vi "自动售货机.vi"() -> ()   [LabVIEW 2011]
panel:
  out "消费额":dbl
  out "投币金额":dbl=79.0
  in  "Tab Control":enum32{"售卖界面", "后台操作界面"}(tab)=enum."后台操作界面"
  out "出货信息":string
  out "显示金额":string
  in  "退币":bool
  in  "5角":bool
  in  "5元":bool
  in  "1元":bool
  in  "10元":bool
  out "果粒橙P":string="0元"
  out "营养快线P":string="0元"
  out "矿泉水P":string="0元"
  out "花生奶P":string="0元"
  out "绿茶P":string="0元"
  out "雪梨P":string="0元"
  in  "果粒橙":bool
  in  "营养快线":bool
  in  "矿泉水":bool
  in  "花生奶":bool
  in  "绿茶":bool
  in  "雪梨":bool
  out "红牛P":string="0元"
  out "八宝粥P":string="0元"
  out "王老吉P":string="0元"
  out "可乐P":string="0元"
  out "雪碧P":string="0元"
  out "百事P":string="0元"
  in  "红牛":bool
  in  "八宝粥":bool
  in  "王老吉":bool
  in  "可乐":bool
  in  "雪碧":bool
  in  "百事":bool
  in  "上货":bool
  in  "关闭售货机":bool
  in  "果粒橙单价":dbl=4.0
  in  "营养快线单价":dbl=3.5
  in  "矿泉水单价":dbl=1.5
  in  "花生奶单价":dbl=3.5
  in  "绿茶单价":dbl=2.5
  in  "雪梨单价":dbl=2.5
  in  "红牛单价":dbl=4.0
  in  "八宝粥单价":dbl=3.0
  in  "王老吉单价":dbl=3.0
  in  "可乐单价":dbl=2.0
  in  "雪碧单价":dbl=2.0
  in  "百事单价":dbl=2.0
  out "销售记录":string
  out "销售金额":string
  in  "果粒橙数量":i32=20
  in  "营养快线数量":i32=20
  in  "矿泉水数量":i32=20
  in  "花生奶数量":i32=20
  in  "绿茶数量":i32=20
  in  "雪梨数量":i32=20
  in  "红牛数量":i32=20
  in  "八宝粥数量":i32=20
  in  "王老吉数量":i32=20
  in  "可乐数量":i32=20
  in  "雪碧数量":i32=20
  in  "百事数量":i32=20
  # "实验中心"
  # "chn"
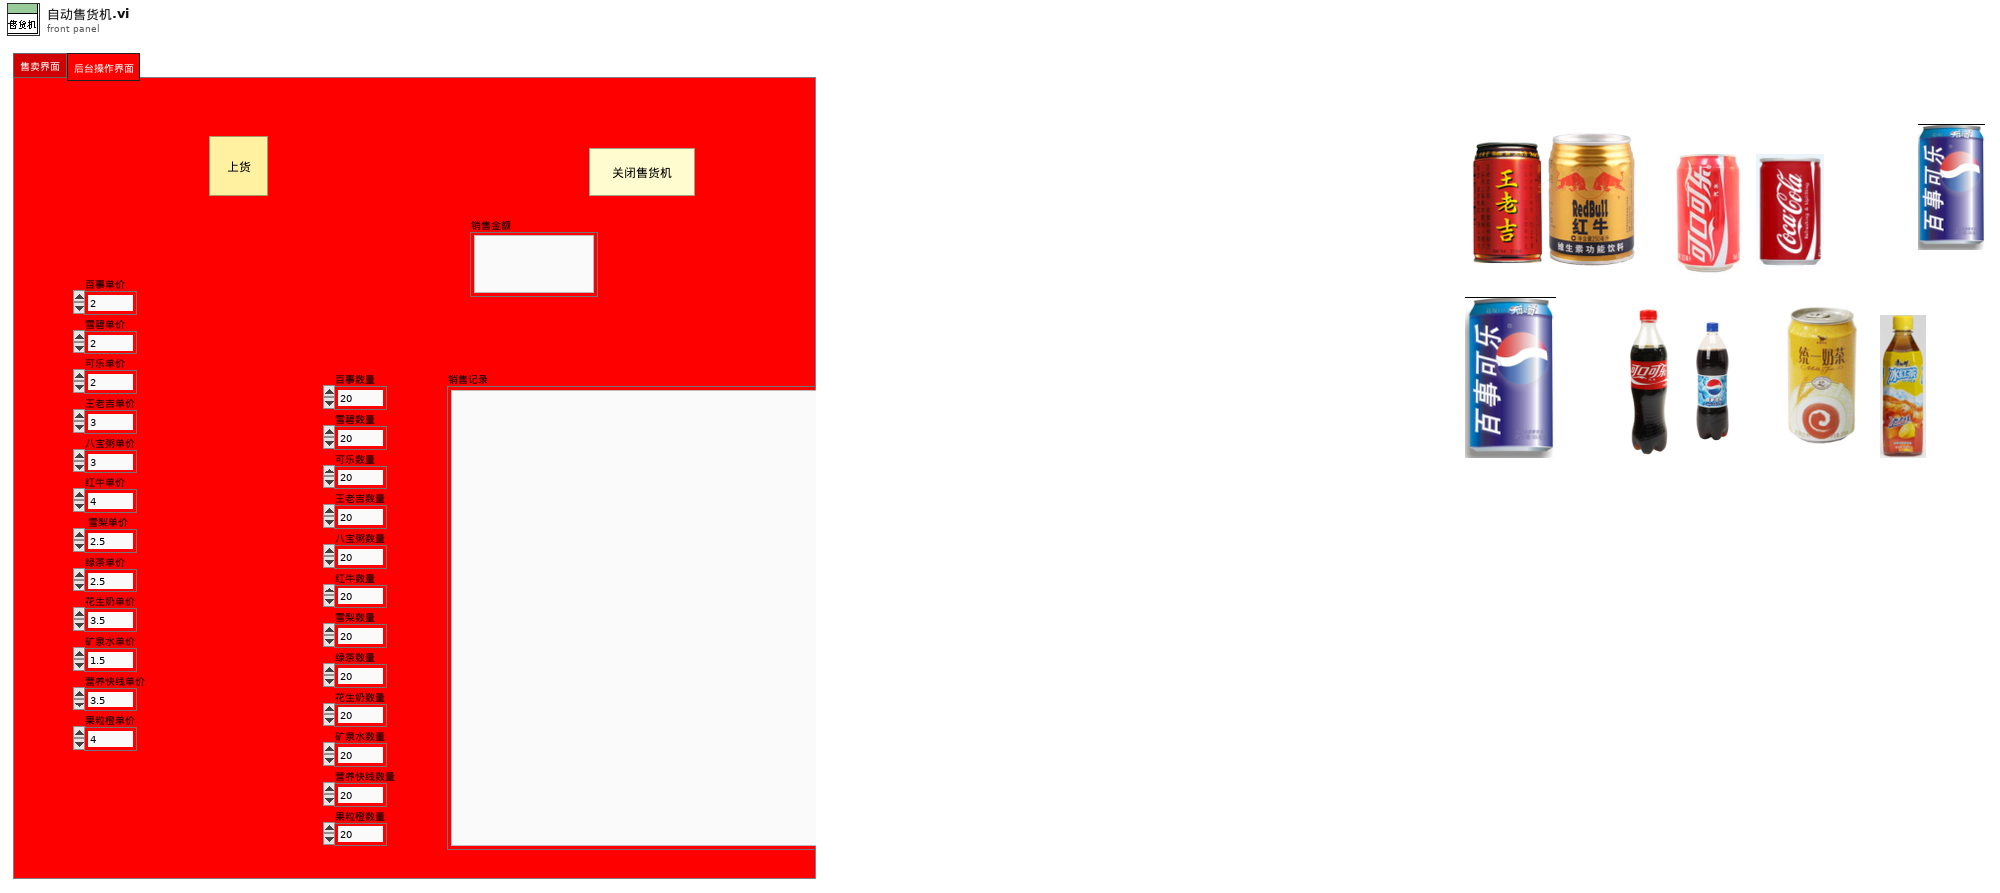
[diagram p1: front panel]
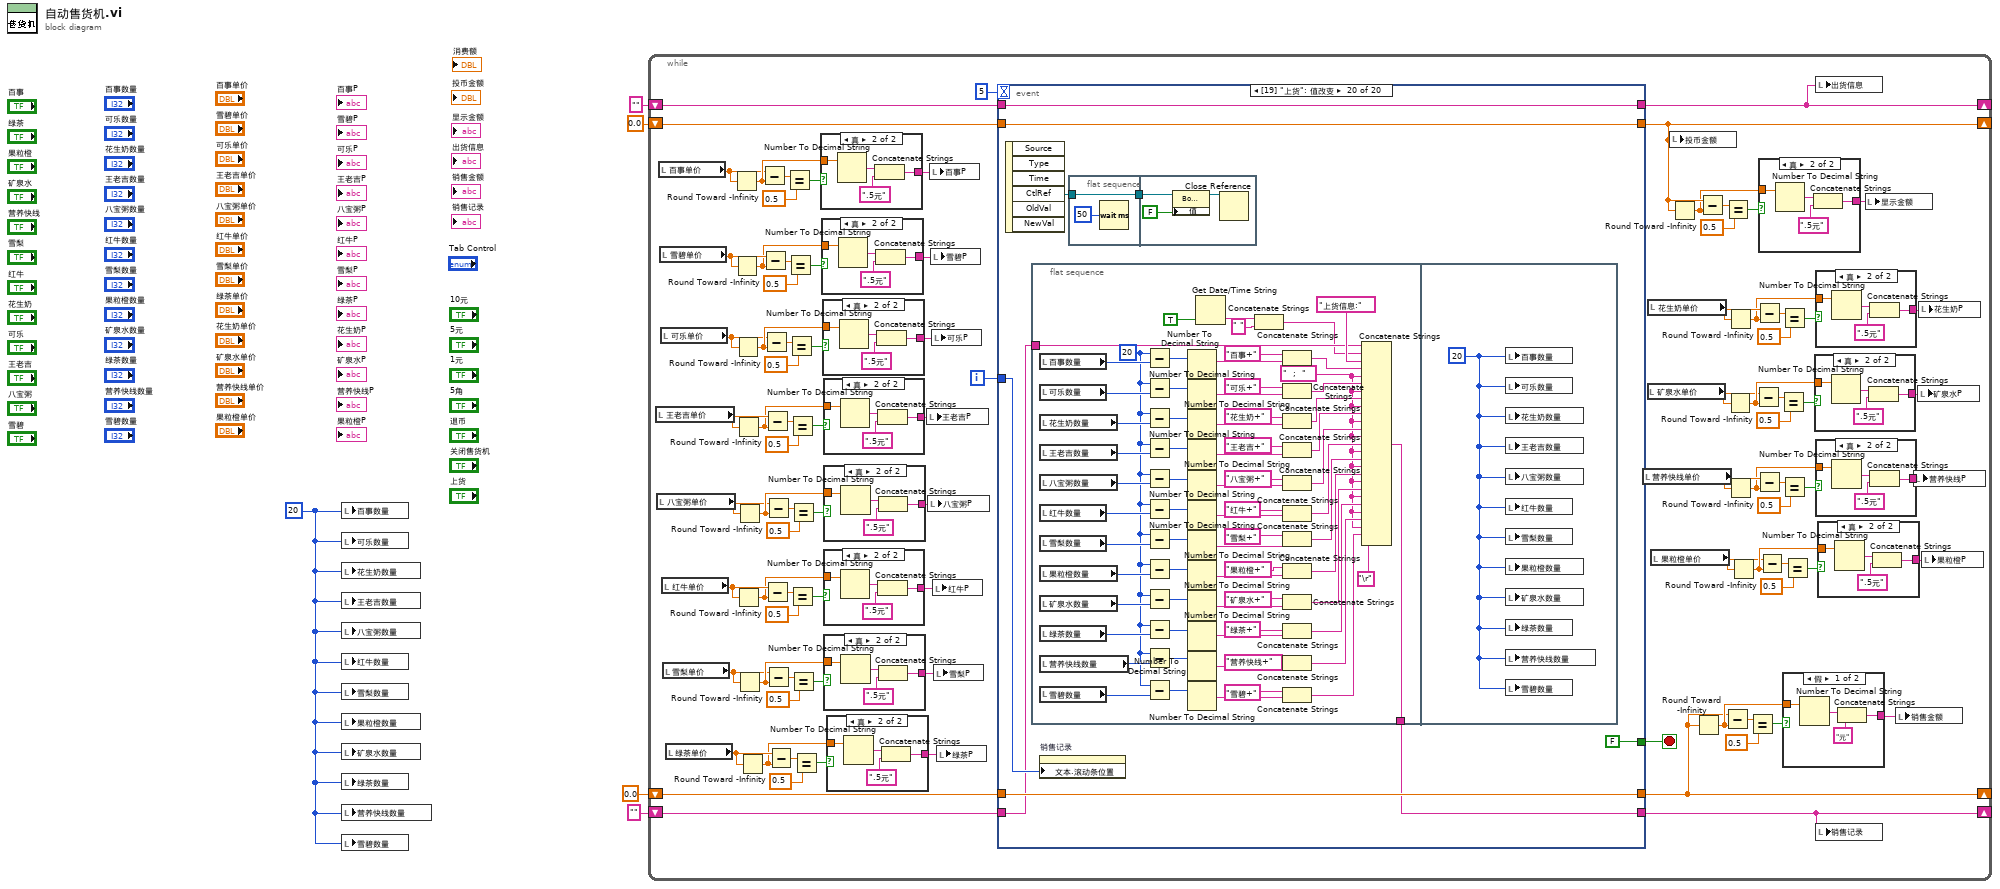
[diagram p0: block diagram]
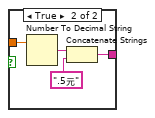
[diagram p2: hidden frame]
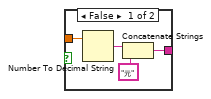
[diagram p3: hidden frame]
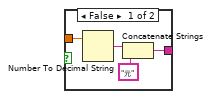
[diagram p4: hidden frame]
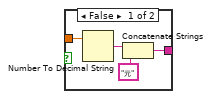
[diagram p5: hidden frame]
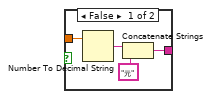
[diagram p6: hidden frame]
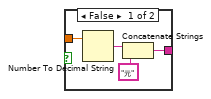
[diagram p7: hidden frame]
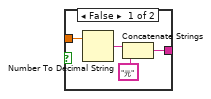
[diagram p8: hidden frame]
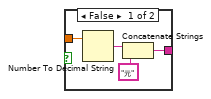
[diagram p9: hidden frame]
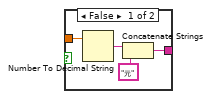
[diagram p10: hidden frame]
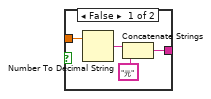
[diagram p11: hidden frame]
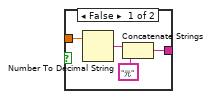
[diagram p12: hidden frame]
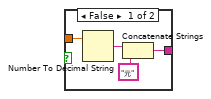
[diagram p13: hidden frame]
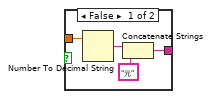
[diagram p14: hidden frame]
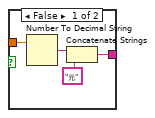
[diagram p15: hidden frame]
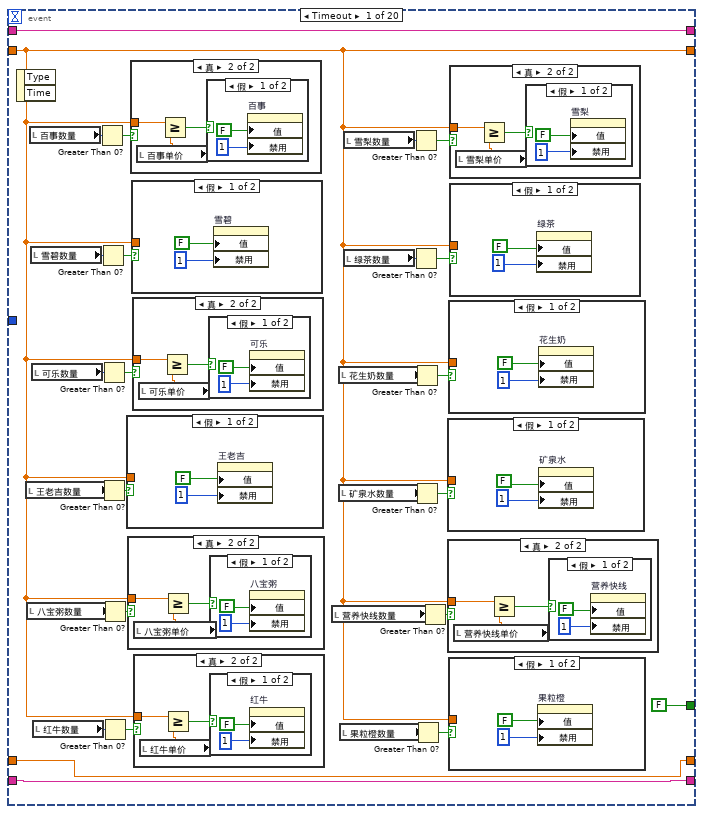
[diagram p16: hidden frame]
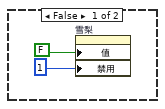
[diagram p17: hidden frame]
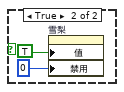
[diagram p18: hidden frame]
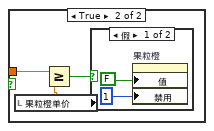
[diagram p19: hidden frame]
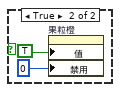
[diagram p20: hidden frame]
diagram:
  w1 = 20 ("百事数量")
  n1 = local write "百事数量"(w1) -> ()
  n2 = local write "可乐数量"(w1) -> ()
  n3 = local write "花生奶数量"(w1) -> ()
  n4 = local write "王老吉数量"(w1) -> ()
  n5 = local write "八宝粥数量"(w1) -> ()
  n6 = local write "红牛数量"(w1) -> ()
  n7 = local write "雪梨数量"(w1) -> ()
  n8 = local write "果粒橙数量"(w1) -> ()
  n9 = local write "矿泉水数量"(w1) -> ()
  n10 = local write "绿茶数量"(w1) -> ()
  n11 = local write "营养快线数量"(w1) -> ()
  n12 = local write "雪碧数量"(w1) -> ()
  n13 = while {
    shift-right: [w92] -> _
    shift-left: 0.0 -> [w98]
    shift-right: [w17] -> _
    shift-left: "" ("出货信息") -> [w16]
    shift-right: [w10] -> _
    shift-left: 0.0 ("消费额") -> [w15]
    shift-right: [w7] -> _
    shift-left: "" ("出货信息") -> [w8]
    i -> [w6]
    stop <- w96 stop-if-true
    n14 = local read "王老吉单价"() -> (w70:dbl)
    n15 = local read "八宝粥单价"() -> (w61:dbl)
    n16 = local read "百事单价"() -> (w85:dbl)
    n17 = local read "雪碧单价"() -> (w82:dbl)
    n18 = local read "可乐单价"() -> (w73:dbl)
    n19 = local read "红牛单价"() -> (w58:dbl)
    n20 = local read "雪梨单价"() -> (w49:dbl)
    n21 = local read "绿茶单价"() -> (w46:dbl)
    n22 = Round Toward -Infinity(1:w85) -> (0:w89:dbl)
    n23 = Round Toward -Infinity(1:w82) -> (0:w78:dbl)
    n24 = Round Toward -Infinity(1:w73) -> (0:w77:dbl)
    n25 = Round Toward -Infinity(1:w70) -> (0:w66:dbl)
    n26 = Round Toward -Infinity(1:w58) -> (0:w54:dbl)
    n27 = Round Toward -Infinity(1:w61) -> (0:w65:dbl)
    n28 = Round Toward -Infinity(1:w49) -> (0:w53:dbl)
    n29 = Round Toward -Infinity(1:w46) -> (0:w42:dbl)
    n30 = Subtract(x=w85, y=w89) -> (x-y=w87:dbl)
    n31 = Subtract(x=w82, y=w78) -> (x-y=w80:dbl)
    n32 = Subtract(x=w73, y=w77) -> (x-y=w75:dbl)
    n33 = Subtract(x=w70, y=w66) -> (x-y=w68:dbl)
    n34 = Subtract(x=w58, y=w54) -> (x-y=w56:dbl)
    n35 = Subtract(x=w61, y=w65) -> (x-y=w63:dbl)
    n36 = Subtract(x=w49, y=w53) -> (x-y=w51:dbl)
    n37 = Subtract(x=w46, y=w42) -> (x-y=w44:dbl)
    n38 = Equal?(x=w87, y=0.5) -> (x = y?=w88:bool)
    n39 = Equal?(x=w80, y=0.5) -> (x = y?=w79:bool)
    n40 = Equal?(x=w75, y=0.5) -> (x = y?=w76:bool)
    n41 = Equal?(x=w68, y=0.5) -> (x = y?=w67:bool)
    n42 = Equal?(x=w56, y=0.5) -> (x = y?=w55:bool)
    n43 = Equal?(x=w63, y=0.5) -> (x = y?=w64:bool)
    n44 = Equal?(x=w51, y=0.5) -> (x = y?=w52:bool)
    n45 = Equal?(x=w44, y=0.5) -> (x = y?=w43:bool)
    n46 = case shown="真" w88 {
      tunnel: w89 -> [w196 w201]
      tunnel: [w195 w199] -> w84
      frame False {
        n47 = Number To Decimal String(number=w196) -> (decimal integer string=w197:string)  [unwired: 1 in]
        n48 = Concatenate Strings(w197, "元" ("string")) -> (w195:string)
      }
      frame True {
        n49 = Number To Decimal String(number=w201) -> (decimal integer string=w202:string)  [unwired: 1 in]
        n50 = Concatenate Strings(w202, ".5元" ("string")) -> (w199:string)
      }
    }
    n51 = case shown="真" w79 {
      tunnel: w78 -> [w188 w193]
      tunnel: [w187 w191] -> w83
      frame False {
        n52 = Number To Decimal String(number=w188) -> (decimal integer string=w189:string)  [unwired: 1 in]
        n53 = Concatenate Strings(w189, "元" ("string")) -> (w187:string)
      }
      frame True {
        n54 = Number To Decimal String(number=w193) -> (decimal integer string=w194:string)  [unwired: 1 in]
        n55 = Concatenate Strings(w194, ".5元" ("string")) -> (w191:string)
      }
    }
    n56 = case shown="真" w76 {
      tunnel: w77 -> [w180 w185]
      tunnel: [w179 w183] -> w72
      frame False {
        n57 = Number To Decimal String(number=w180) -> (decimal integer string=w181:string)  [unwired: 1 in]
        n58 = Concatenate Strings(w181, "元" ("string")) -> (w179:string)
      }
      frame True {
        n59 = Number To Decimal String(number=w185) -> (decimal integer string=w186:string)  [unwired: 1 in]
        n60 = Concatenate Strings(w186, ".5元" ("string")) -> (w183:string)
      }
    }
    n61 = case shown="真" w67 {
      tunnel: w66 -> [w172 w177]
      tunnel: [w171 w175] -> w71
      frame False {
        n62 = Number To Decimal String(number=w172) -> (decimal integer string=w173:string)  [unwired: 1 in]
        n63 = Concatenate Strings(w173, "元" ("string")) -> (w171:string)
      }
      frame True {
        n64 = Number To Decimal String(number=w177) -> (decimal integer string=w178:string)  [unwired: 1 in]
        n65 = Concatenate Strings(w178, ".5元" ("string")) -> (w175:string)
      }
    }
    n66 = case shown="真" w55 {
      tunnel: w54 -> [w156 w161]
      tunnel: [w155 w159] -> w59
      frame False {
        n67 = Number To Decimal String(number=w156) -> (decimal integer string=w157:string)  [unwired: 1 in]
        n68 = Concatenate Strings(w157, "元" ("string")) -> (w155:string)
      }
      frame True {
        n69 = Number To Decimal String(number=w161) -> (decimal integer string=w162:string)  [unwired: 1 in]
        n70 = Concatenate Strings(w162, ".5元" ("string")) -> (w159:string)
      }
    }
    n71 = case shown="真" w64 {
      tunnel: w65 -> [w164 w169]
      tunnel: [w163 w167] -> w60
      frame False {
        n72 = Number To Decimal String(number=w164) -> (decimal integer string=w165:string)  [unwired: 1 in]
        n73 = Concatenate Strings(w165, "元" ("string")) -> (w163:string)
      }
      frame True {
        n74 = Number To Decimal String(number=w169) -> (decimal integer string=w170:string)  [unwired: 1 in]
        n75 = Concatenate Strings(w170, ".5元" ("string")) -> (w167:string)
      }
    }
    n76 = case shown="真" w52 {
      tunnel: w53 -> [w148 w153]
      tunnel: [w147 w151] -> w48
      frame False {
        n77 = Number To Decimal String(number=w148) -> (decimal integer string=w149:string)  [unwired: 1 in]
        n78 = Concatenate Strings(w149, "元" ("string")) -> (w147:string)
      }
      frame True {
        n79 = Number To Decimal String(number=w153) -> (decimal integer string=w154:string)  [unwired: 1 in]
        n80 = Concatenate Strings(w154, ".5元" ("string")) -> (w151:string)
      }
    }
    n81 = case shown="真" w43 {
      tunnel: w42 -> [w140 w145]
      tunnel: [w139 w143] -> w47
      frame False {
        n82 = Number To Decimal String(number=w140) -> (decimal integer string=w141:string)  [unwired: 1 in]
        n83 = Concatenate Strings(w141, "元" ("string")) -> (w139:string)
      }
      frame True {
        n84 = Number To Decimal String(number=w145) -> (decimal integer string=w146:string)  [unwired: 1 in]
        n85 = Concatenate Strings(w146, ".5元" ("string")) -> (w143:string)
      }
    }
    n86 = local write "王老吉P"(w71) -> ()
    n87 = local write "八宝粥P"(w60) -> ()
    n88 = local write "百事P"(w84) -> ()
    n89 = local write "雪碧P"(w83) -> ()
    n90 = local write "可乐P"(w72) -> ()
    n91 = local write "红牛P"(w59) -> ()
    n92 = local write "雪梨P"(w48) -> ()
    n93 = local write "绿茶P"(w47) -> ()
    n94 = event shown="[19] \"上货\": 值改变" {
      selector: _ -> [_ _ _ _ _ _ _ _ _ _ _ _ _ _ _ _ _ _ _ _]
      dyn-events: _ -> [_ _ _ _ _ _ _ _ _ _ _ _ _ _ _ _ _ _ _ _]
      timeout: 5 -> [_ _ _ _ _ _ _ _ _ _ _ _ _ _ _ _ _ _ _ _]
      tunnel: [w214 w362 w382 w406 w428 0.0 0.0 w503 w537 w570 w603 w636 w670 w703 w737 w769 w803 w835 w867 w882] -> w92
      tunnel: w98 -> [w214 w364 w383 w407 w429 _ w457 w504 w539 w571 w604 w637 w669 w702 w735 w768 w802 w834 w868 w882]
      tunnel: [FALSE ("Value") FALSE ("Value") FALSE ("Value") FALSE ("Value") FALSE ("Value") TRUE ("Value") FALSE ("Value") FALSE ("Value") FALSE ("Value") FALSE ("Value") FALSE ("Value") FALSE ("Value") FALSE ("Value") FALSE ("Value") FALSE ("Value") FALSE ("Value") FALSE ("Value") FALSE ("Value") FALSE ("Value") FALSE ("Value")] -> w96
      tunnel: w16 -> [w213 w357 w379 w401 w423 w439 w454 w498 w530 w563 w596 w629 w662 w695 w728 w761 w794 w827 w860 w883]
      tunnel: [w213 w358 w380 w402 w424 w439 w453 w497 w531 w564 w597 w630 w663 w696 w729 w762 w795 w828 w861 w883] -> w17
      tunnel: w15 -> [w212 w350 w372 w394 w416 w438 w447 w490 w523 w556 w589 w622 w655 w688 w721 w754 w787 w820 w853 w881]
      tunnel: [w212 w350 w372 w394 w416 w438 w447 w488 w521 w554 w587 w620 w653 w686 w712 w752 w785 w818 w851 w881] -> w10
      tunnel: w8 -> [w211 w349 w371 w393 w415 w437 w446 w481 w515 w548 w581 w614 w647 w680 w714 w746 w779 w812 w845 w875]
      tunnel: [w211 w349 w371 w393 w415 w437 w446 w480 w514 w546 w580 w613 w646 w679 w713 w745 w778 w811 w844 w877] -> w7
      tunnel: w6 -> [_ w348 w370 w392 w414 _ w445 w479 w512 w545 w578 w611 w644 w677 w710 w743 w776 w809 w842 w876]
      event Timeout {
        n95 = event-data() -> ()  [unwired: 1 in, 2 out]
        n96 = local read "王老吉数量"() -> (w231:i32)
        n97 = local read "八宝粥数量"() -> (w227:i32)
        n98 = local read "百事数量"() -> (w238:i32)
        n99 = local read "雪碧数量"() -> (w235:i32)
        n100 = local read "可乐数量"() -> (w234:i32)
        n101 = local read "红牛数量"() -> (w230:i32)
        n102 = Greater Than 0?(x=w238) -> (x > 0?=w237:bool)
        n103 = Greater Than 0?(x=w235) -> (x > 0?=w236:bool)
        n104 = Greater Than 0?(x=w234) -> (x > 0?=w233:bool)
        n105 = Greater Than 0?(x=w231) -> (x > 0?=w232:bool)
        n106 = Greater Than 0?(x=w227) -> (x > 0?=w228:bool)
        n107 = Greater Than 0?(x=w230) -> (x > 0?=w229:bool)
        n108 = case shown="假" w232 {
          tunnel: w214 -> [_ w316]
          frame False {
            n109 = property on="王老吉" class="Bool (严格)"("值"=FALSE ("百事"), "禁用"=u8 1 ("Disabled")) -> ()  [unwired: 2 in, 2 out]
          }
          frame True {
            n110 = local read "王老吉单价"() -> (w315:dbl)
            n111 = Greater Or Equal?(x=w316, y=w315) -> (x >= y?=w314:bool)
            n112 = case shown="假" w314 {
              frame False {
                n113 = property on="王老吉" class="Bool (严格)"("值"=FALSE ("百事"), "禁用"=u8 1 ("Disabled")) -> ()  [unwired: 2 in, 2 out]
              }
              frame True {
                n114 = property on="王老吉" class="Bool (严格)"("值"=TRUE ("百事"), "禁用"=u8 0 ("Disabled")) -> ()  [unwired: 2 in, 2 out]
              }
            }
          }
        }
        n115 = case shown="真" w228 {
          tunnel: w214 -> [_ w307]
          frame False {
            n116 = property on="八宝粥" class="Bool (严格)"("值"=FALSE ("百事"), "禁用"=u8 1 ("Disabled")) -> ()  [unwired: 2 in, 2 out]
          }
          frame True {
            n117 = local read "八宝粥单价"() -> (w306:dbl)
            n118 = Greater Or Equal?(x=w307, y=w306) -> (x >= y?=w305:bool)
            n119 = case shown="假" w305 {
              frame False {
                n120 = property on="八宝粥" class="Bool (严格)"("值"=FALSE ("百事"), "禁用"=u8 1 ("Disabled")) -> ()  [unwired: 2 in, 2 out]
              }
              frame True {
                n121 = property on="八宝粥" class="Bool (严格)"("值"=TRUE ("百事"), "禁用"=u8 0 ("Disabled")) -> ()  [unwired: 2 in, 2 out]
              }
            }
          }
        }
        n122 = case shown="真" w237 {
          tunnel: w214 -> [_ w343]
          frame False {
            n123 = property on="百事" class="Bool (严格)"("值"=FALSE ("百事"), "禁用"=u8 1 ("Disabled")) -> ()  [unwired: 2 in, 2 out]
          }
          frame True {
            n124 = local read "百事单价"() -> (w342:dbl)
            n125 = Greater Or Equal?(x=w343, y=w342) -> (x >= y?=w341:bool)
            n126 = case shown="假" w341 {
              frame False {
                n127 = property on="百事" class="Bool (严格)"("值"=FALSE ("百事"), "禁用"=u8 1 ("Disabled")) -> ()  [unwired: 2 in, 2 out]
              }
              frame True {
                n128 = property on="百事" class="Bool (严格)"("值"=TRUE ("百事"), "禁用"=u8 0 ("Disabled")) -> ()  [unwired: 2 in, 2 out]
              }
            }
          }
        }
        n129 = case shown="假" w236 {
          tunnel: w214 -> [_ w334]
          frame False {
            n130 = property on="雪碧" class="Bool (严格)"("值"=FALSE ("百事"), "禁用"=u8 1 ("Disabled")) -> ()  [unwired: 2 in, 2 out]
          }
          frame True {
            n131 = local read "雪碧单价"() -> (w333:dbl)
            n132 = Greater Or Equal?(x=w334, y=w333) -> (x >= y?=w332:bool)
            n133 = case shown="假" w332 {
              frame False {
                n134 = property on="雪碧" class="Bool (严格)"("值"=FALSE ("百事"), "禁用"=u8 1 ("Disabled")) -> ()  [unwired: 2 in, 2 out]
              }
              frame True {
                n135 = property on="雪碧" class="Bool (严格)"("值"=TRUE ("百事"), "禁用"=u8 0 ("Disabled")) -> ()  [unwired: 2 in, 2 out]
              }
            }
          }
        }
        n136 = case shown="真" w233 {
          tunnel: w214 -> [_ w325]
          frame False {
            n137 = property on="可乐" class="Bool (严格)"("值"=FALSE ("百事"), "禁用"=u8 1 ("Disabled")) -> ()  [unwired: 2 in, 2 out]
          }
          frame True {
            n138 = local read "可乐单价"() -> (w324:dbl)
            n139 = Greater Or Equal?(x=w325, y=w324) -> (x >= y?=w323:bool)
            n140 = case shown="假" w323 {
              frame False {
                n141 = property on="可乐" class="Bool (严格)"("值"=FALSE ("百事"), "禁用"=u8 1 ("Disabled")) -> ()  [unwired: 2 in, 2 out]
              }
              frame True {
                n142 = property on="可乐" class="Bool (严格)"("值"=TRUE ("百事"), "禁用"=u8 0 ("Disabled")) -> ()  [unwired: 2 in, 2 out]
              }
            }
          }
        }
        n143 = case shown="真" w229 {
          tunnel: w214 -> [_ w298]
          frame False {
            n144 = property on="红牛" class="Bool (严格)"("值"=FALSE ("百事"), "禁用"=u8 1 ("Disabled")) -> ()  [unwired: 2 in, 2 out]
          }
          frame True {
            n145 = local read "红牛单价"() -> (w297:dbl)
            n146 = Greater Or Equal?(x=w298, y=w297) -> (x >= y?=w296:bool)
            n147 = case shown="假" w296 {
              frame False {
                n148 = property on="红牛" class="Bool (严格)"("值"=FALSE ("百事"), "禁用"=u8 1 ("Disabled")) -> ()  [unwired: 2 in, 2 out]
              }
              frame True {
                n149 = property on="红牛" class="Bool (严格)"("值"=TRUE ("百事"), "禁用"=u8 0 ("Disabled")) -> ()  [unwired: 2 in, 2 out]
              }
            }
          }
        }
        n150 = local read "营养快线数量"() -> (w226:i32)
        n151 = local read "花生奶数量"() -> (w219:i32)
        n152 = local read "矿泉水数量"() -> (w222:i32)
        n153 = local read "果粒橙数量"() -> (w223:i32)
        n154 = local read "雪梨数量"() -> (w215:i32)
        n155 = local read "绿茶数量"() -> (w218:i32)
        n156 = Greater Than 0?(x=w215) -> (x > 0?=w216:bool)
        n157 = Greater Than 0?(x=w218) -> (x > 0?=w217:bool)
        n158 = Greater Than 0?(x=w219) -> (x > 0?=w220:bool)
        n159 = Greater Than 0?(x=w222) -> (x > 0?=w221:bool)
        n160 = Greater Than 0?(x=w223) -> (x > 0?=w224:bool)
        n161 = Greater Than 0?(x=w226) -> (x > 0?=w225:bool)
        n162 = case shown="假" w221 {
          tunnel: w214 -> [_ w271]
          frame False {
            n163 = property on="矿泉水" class="Bool (严格)"("值"=FALSE ("百事"), "禁用"=u8 1 ("Disabled")) -> ()  [unwired: 2 in, 2 out]
          }
          frame True {
            n164 = local read "矿泉水单价"() -> (w270:dbl)
            n165 = Greater Or Equal?(x=w271, y=w270) -> (x >= y?=w269:bool)
            n166 = case shown="假" w269 {
              frame False {
                n167 = property on="矿泉水" class="Bool (严格)"("值"=FALSE ("百事"), "禁用"=u8 1 ("Disabled")) -> ()  [unwired: 2 in, 2 out]
              }
              frame True {
                n168 = property on="矿泉水" class="Bool (严格)"("值"=TRUE ("百事"), "禁用"=u8 0 ("Disabled")) -> ()  [unwired: 2 in, 2 out]
              }
            }
          }
        }
        n169 = case shown="真" w225 {
          tunnel: w214 -> [_ w262]
          frame False {
            n170 = property on="营养快线" class="Bool (严格)"("值"=FALSE ("百事"), "禁用"=u8 1 ("Disabled")) -> ()  [unwired: 2 in, 2 out]
          }
          frame True {
            n171 = local read "营养快线单价"() -> (w261:dbl)
            n172 = Greater Or Equal?(x=w262, y=w261) -> (x >= y?=w260:bool)
            n173 = case shown="假" w260 {
              frame False {
                n174 = property on="营养快线" class="Bool (严格)"("值"=FALSE ("百事"), "禁用"=u8 1 ("Disabled")) -> ()  [unwired: 2 in, 2 out]
              }
              frame True {
                n175 = property on="营养快线" class="Bool (严格)"("值"=TRUE ("百事"), "禁用"=u8 0 ("Disabled")) -> ()  [unwired: 2 in, 2 out]
              }
            }
          }
        }
        n176 = case shown="假" w220 {
          tunnel: w214 -> [_ w280]
          frame False {
            n177 = property on="花生奶" class="Bool (严格)"("值"=FALSE ("百事"), "禁用"=u8 1 ("Disabled")) -> ()  [unwired: 2 in, 2 out]
          }
          frame True {
            n178 = local read "花生奶单价"() -> (w279:dbl)
            n179 = Greater Or Equal?(x=w280, y=w279) -> (x >= y?=w278:bool)
            n180 = case shown="假" w278 {
              frame False {
                n181 = property on="花生奶" class="Bool (严格)"("值"=FALSE ("百事"), "禁用"=u8 1 ("Disabled")) -> ()  [unwired: 2 in, 2 out]
              }
              frame True {
                n182 = property on="花生奶" class="Bool (严格)"("值"=TRUE ("百事"), "禁用"=u8 0 ("Disabled")) -> ()  [unwired: 2 in, 2 out]
              }
            }
          }
        }
        n183 = case shown="假" w224 {
          tunnel: w214 -> [_ w253]
          frame False {
            n184 = property on="果粒橙" class="Bool (严格)"("值"=FALSE ("百事"), "禁用"=u8 1 ("Disabled")) -> ()  [unwired: 2 in, 2 out]
          }
          frame True {
            n185 = local read "果粒橙单价"() -> (w252:dbl)
            n186 = Greater Or Equal?(x=w253, y=w252) -> (x >= y?=w251:bool)
            n187 = case shown="假" w251 {
              frame False {
                n188 = property on="果粒橙" class="Bool (严格)"("值"=FALSE ("百事"), "禁用"=u8 1 ("Disabled")) -> ()  [unwired: 2 in, 2 out]
              }
              frame True {
                n189 = property on="果粒橙" class="Bool (严格)"("值"=TRUE ("百事"), "禁用"=u8 0 ("Disabled")) -> ()  [unwired: 2 in, 2 out]
              }
            }
          }
        }
        n190 = case shown="真" w216 {
          tunnel: w214 -> [_ w244]
          frame False {
            n191 = property on="雪梨" class="Bool (严格)"("值"=FALSE ("百事"), "禁用"=u8 1 ("Disabled")) -> ()  [unwired: 2 in, 2 out]
          }
          frame True {
            n192 = local read "雪梨单价"() -> (w243:dbl)
            n193 = Greater Or Equal?(x=w244, y=w243) -> (x >= y?=w242:bool)
            n194 = case shown="假" w242 {
              frame False {
                n195 = property on="雪梨" class="Bool (严格)"("值"=FALSE ("百事"), "禁用"=u8 1 ("Disabled")) -> ()  [unwired: 2 in, 2 out]
              }
              frame True {
                n196 = property on="雪梨" class="Bool (严格)"("值"=TRUE ("百事"), "禁用"=u8 0 ("Disabled")) -> ()  [unwired: 2 in, 2 out]
              }
            }
          }
        }
        n197 = case shown="假" w217 {
          tunnel: w214 -> [_ w289]
          frame False {
            n198 = property on="绿茶" class="Bool (严格)"("值"=FALSE ("百事"), "禁用"=u8 1 ("Disabled")) -> ()  [unwired: 2 in, 2 out]
          }
          frame True {
            n199 = local read "绿茶单价"() -> (w288:dbl)
            n200 = Greater Or Equal?(x=w289, y=w288) -> (x >= y?=w287:bool)
            n201 = case shown="假" w287 {
              frame False {
                n202 = property on="绿茶" class="Bool (严格)"("值"=FALSE ("百事"), "禁用"=u8 1 ("Disabled")) -> ()  [unwired: 2 in, 2 out]
              }
              frame True {
                n203 = property on="绿茶" class="Bool (严格)"("值"=TRUE ("百事"), "禁用"=u8 0 ("Disabled")) -> ()  [unwired: 2 in, 2 out]
              }
            }
          }
        }
      }
      event "10元": Value Change {
        n204 = event-data() -> ("CtlRef"=w360:refnum<vi>)  [unwired: 1 in, 5 out]
        n205 = property on="出货信息" class="Str"("文本.滚动条位置"=w348) -> ()  [unwired: 2 in, 2 out]
        n206 = flat-sequence {
          tunnel: [w366] -> w361
          tunnel: w360 -> [w366]
          tunnel: w361 -> [w369]
          frame #0 {
            n207 = Wait (ms)(milliseconds to wait=u32 50) -> ()  [unwired: 1 out]
          }
          frame #1 {
            n208 = property class="Bool (strict)"(reference=w369, "值"=FALSE ("Value")) -> (reference out=w367:refnum<vi>)  [unwired: 1 in, 1 out]
            n209 = Close Reference(reference=w367) -> ()  [unwired: 1 in, 1 out]
          }
        }
        n210 = Get Date/Time String(want seconds? (F)=TRUE) -> (time string=w353:string)  [unwired: 2 in, 1 out]
        n211 = Concatenate Strings(w353, " " ("string")) -> (w351:string)
        n212 = Concatenate Strings(w357, w351, "投币 ￥：10元！" ("出货信息"), "\r") -> (w358:string)
        n213 = Add(x=w364, y=10.0) -> (x+y=w362:dbl)
      }
      event "5元": Value Change {
        n214 = event-data() -> ("CtlRef"=w385:refnum<vi>)  [unwired: 1 in, 5 out]
        n215 = property on="出货信息" class="Str"("文本.滚动条位置"=w370) -> ()  [unwired: 2 in, 2 out]
        n216 = flat-sequence {
          tunnel: [w388] -> w386
          tunnel: w385 -> [w388]
          tunnel: w386 -> [w391]
          frame #0 {
            n217 = Wait (ms)(milliseconds to wait=u32 50) -> ()  [unwired: 1 out]
          }
          frame #1 {
            n218 = property class="Bool (strict)"(reference=w391, "值"=FALSE ("Value")) -> (reference out=w389:refnum<vi>)  [unwired: 1 in, 1 out]
            n219 = Close Reference(reference=w389) -> ()  [unwired: 1 in, 1 out]
          }
        }
        n220 = Get Date/Time String(want seconds? (F)=TRUE) -> (time string=w375:string)  [unwired: 2 in, 1 out]
        n221 = Concatenate Strings(w375, " " ("string")) -> (w373:string)
        n222 = Concatenate Strings(w379, w373, "投币 ￥：5元！" ("出货信息"), "\r") -> (w380:string)
        n223 = Add(x=w383, y=5.0) -> (x+y=w382:dbl)
      }
      event "1元": Value Change {
        n224 = event-data() -> ("CtlRef"=w404:refnum<vi>)  [unwired: 1 in, 5 out]
        n225 = property on="出货信息" class="Str"("文本.滚动条位置"=w392) -> ()  [unwired: 2 in, 2 out]
        n226 = flat-sequence {
          tunnel: [w410] -> w405
          tunnel: w404 -> [w410]
          tunnel: w405 -> [w413]
          frame #0 {
            n227 = Wait (ms)(milliseconds to wait=u32 50) -> ()  [unwired: 1 out]
          }
          frame #1 {
            n228 = property class="Bool (strict)"(reference=w413, "值"=FALSE ("Value")) -> (reference out=w411:refnum<vi>)  [unwired: 1 in, 1 out]
            n229 = Close Reference(reference=w411) -> ()  [unwired: 1 in, 1 out]
          }
        }
        n230 = Get Date/Time String(want seconds? (F)=TRUE) -> (time string=w397:string)  [unwired: 2 in, 1 out]
        n231 = Concatenate Strings(w397, " " ("string")) -> (w395:string)
        n232 = Concatenate Strings(w401, w395, "投币 ￥：1元！" ("出货信息"), "\r") -> (w402:string)
        n233 = Add(x=w407, y=1.0) -> (x+y=w406:dbl)
      }
      event "5角": Value Change {
        n234 = event-data() -> ("CtlRef"=w426:refnum<vi>)  [unwired: 1 in, 5 out]
        n235 = property on="出货信息" class="Str"("文本.滚动条位置"=w414) -> ()  [unwired: 2 in, 2 out]
        n236 = flat-sequence {
          tunnel: [w432] -> w427
          tunnel: w426 -> [w432]
          tunnel: w427 -> [w435]
          frame #0 {
            n237 = Wait (ms)(milliseconds to wait=u32 50) -> ()  [unwired: 1 out]
          }
          frame #1 {
            n238 = property class="Bool (strict)"(reference=w435, "值"=FALSE ("Value")) -> (reference out=w433:refnum<vi>)  [unwired: 1 in, 1 out]
            n239 = Close Reference(reference=w433) -> ()  [unwired: 1 in, 1 out]
          }
        }
        n240 = Get Date/Time String(want seconds? (F)=TRUE) -> (time string=w419:string)  [unwired: 2 in, 1 out]
        n241 = Concatenate Strings(w419, " " ("string")) -> (w417:string)
        n242 = Concatenate Strings(w423, w417, "投币 ￥：0.5元！" ("出货信息"), "\r") -> (w424:string)
        n243 = Add(x=w429, y=0.5) -> (x+y=w428:dbl)
      }
      event "关闭售货机": Value Change {
        n244 = event-data() -> ("CtlRef"=w441:refnum<vi>)  [unwired: 1 in, 5 out]
        n245 = property class="Bool (strict)"(reference=w441, "值"=FALSE ("Value")) -> (reference out=w440:refnum<vi>)  [unwired: 1 in, 1 out]
        n246 = Close Reference(reference=w440) -> ()  [unwired: 1 in, 1 out]
        n247 = Quit LabVIEW(quit? (T)=TRUE) -> ()
      }
      event "退币": Value Change {
        n248 = event-data() -> ("CtlRef"=w464:refnum<vi>)  [unwired: 1 in, 5 out]
        n249 = property on="出货信息" class="Str"("文本.滚动条位置"=w445) -> ()  [unwired: 2 in, 2 out]
        n250 = flat-sequence {
          tunnel: [w475] -> w465
          tunnel: w464 -> [w475]
          tunnel: w465 -> [w478]
          frame #0 {
            n251 = Wait (ms)(milliseconds to wait=u32 50) -> ()  [unwired: 1 out]
          }
          frame #1 {
            n252 = property class="Bool (strict)"(reference=w478, "值"=FALSE ("Value")) -> (reference out=w476:refnum<vi>)  [unwired: 1 in, 1 out]
            n253 = Close Reference(reference=w476) -> ()  [unwired: 1 in, 1 out]
          }
        }
        n254 = Round Toward -Infinity(1:w457) -> (0:w461:dbl)
        n255 = Subtract(x=w457, y=w461) -> (x-y=w459:dbl)
        n256 = Equal?(x=w459, y=0.5) -> (x = y?=w460:bool)
        n257 = case shown="假" w460 {
          tunnel: w461 -> [w467 w472]
          tunnel: [w466 w470] -> w456
          frame False {
            n258 = Number To Decimal String(number=w467) -> (decimal integer string=w468:string)  [unwired: 1 in]
            n259 = Concatenate Strings(w468, "元！" ("string")) -> (w466:string)
          }
          frame True {
            n260 = Number To Decimal String(number=w472) -> (decimal integer string=w473:string)  [unwired: 1 in]
            n261 = Concatenate Strings(w473, ".5元！" ("string")) -> (w470:string)
          }
        }
        n262 = Get Date/Time String(want seconds? (F)=TRUE) -> (time string=w450:string)  [unwired: 2 in, 1 out]
        n263 = Concatenate Strings(w450, " " ("string")) -> (w448:string)
        n264 = Concatenate Strings(w454, w448, "退币 ￥：" ("string"), w456, "\r") -> (w453:string)
      }
      event "百事": Value Change {
        n265 = event-data() -> ("CtlRef"=w499:refnum<vi>)  [unwired: 1 in, 5 out]
        n266 = property on="出货信息" class="Str"("文本.滚动条位置"=w479) -> ()  [unwired: 2 in, 2 out]
        n267 = property on="销售记录" class="Str"("文本.滚动条位置"=w479) -> ()  [unwired: 2 in, 2 out]
        n268 = local read "百事单价"() -> (w489:dbl)
        n269 = flat-sequence {
          tunnel: [w508] -> w500
          tunnel: w499 -> [w508]
          tunnel: w500 -> [w511]
          frame #0 {
            n270 = Wait (ms)(milliseconds to wait=u32 50) -> ()  [unwired: 1 out]
          }
          frame #1 {
            n271 = property class="Bool (strict)"(reference=w511, "值"=TRUE ("Value")) -> (reference out=w509:refnum<vi>)  [unwired: 1 in, 1 out]
            n272 = Close Reference(reference=w509) -> ()  [unwired: 1 in, 1 out]
          }
        }
        n273 = Add(x=w489, y=w490) -> (x+y=w488:dbl)
        n274 = local write "消费额"(w488) -> ()
        n275 = local read "百事数量"() -> (w502:i32)
        n276 = Get Date/Time String(want seconds? (F)=TRUE) -> (time string=w493:string)  [unwired: 2 in, 1 out]
        n277 = Decrement(x=w502) -> (x-1=w501:i32)
        n278 = Concatenate Strings(w493, " " ("string")) -> (w491:string)
        n279 = Get Date/Time String(want seconds? (F)=TRUE) -> (time string=w486:string)  [unwired: 2 in, 1 out]
        n280 = local write "百事数量"(w501) -> ()
        n281 = Concatenate Strings(w486, " " ("string")) -> (w482:string)
        n282 = Concatenate Strings(w481, w482, "百事可乐1罐！" ("出货信息"), "\r") -> (w480:string)
        n283 = Concatenate Strings(w498, w491, "百事可乐1罐！" ("出货信息"), "\r") -> (w497:string)
        n284 = local read "百事单价"() -> (w505:dbl)
        n285 = Subtract(x=w504, y=w505) -> (x-y=w503:dbl)
      }
      event "雪碧": Value Change {
        n286 = event-data() -> ("CtlRef"=w533:refnum<vi>)  [unwired: 1 in, 5 out]
        n287 = property on="出货信息" class="Str"("文本.滚动条位置"=w512) -> ()  [unwired: 2 in, 2 out]
        n288 = property on="销售记录" class="Str"("文本.滚动条位置"=w512) -> ()  [unwired: 2 in, 2 out]
        n289 = local read "雪碧单价"() -> (w522:dbl)
        n290 = flat-sequence {
          tunnel: [w541] -> w534
          tunnel: w533 -> [w541]
          tunnel: w534 -> [w544]
          frame #0 {
            n291 = Wait (ms)(milliseconds to wait=u32 50) -> ()  [unwired: 1 out]
          }
          frame #1 {
            n292 = property class="Bool (strict)"(reference=w544, "值"=TRUE ("Value")) -> (reference out=w542:refnum<vi>)  [unwired: 1 in, 1 out]
            n293 = Close Reference(reference=w542) -> ()  [unwired: 1 in, 1 out]
          }
        }
        n294 = Add(x=w522, y=w523) -> (x+y=w521:dbl)
        n295 = local write "消费额"(w521) -> ()
        n296 = Get Date/Time String(want seconds? (F)=TRUE) -> (time string=w526:string)  [unwired: 2 in, 1 out]
        n297 = local read "雪碧数量"() -> (w536:i32)
        n298 = Concatenate Strings(w526, " " ("string")) -> (w524:string)
        n299 = Get Date/Time String(want seconds? (F)=TRUE) -> (time string=w519:string)  [unwired: 2 in, 1 out]
        n300 = Decrement(x=w536) -> (x-1=w535:i32)
        n301 = local write "雪碧数量"(w535) -> ()
        n302 = Concatenate Strings(w519, " " ("string")) -> (w516:string)
        n303 = Concatenate Strings(w530, w524, "雪碧1罐！" ("出货信息"), "\r") -> (w531:string)
        n304 = Concatenate Strings(w515, w516, "雪碧1罐！" ("出货信息"), "\r") -> (w514:string)
        n305 = local read "雪碧单价"() -> (w538:dbl)
        n306 = Subtract(x=w539, y=w538) -> (x-y=w537:dbl)
      }
      event "可乐": Value Change {
        n307 = event-data() -> ("CtlRef"=w568:refnum<vi>)  [unwired: 1 in, 5 out]
        n308 = property on="出货信息" class="Str"("文本.滚动条位置"=w545) -> ()  [unwired: 2 in, 2 out]
        n309 = property on="销售记录" class="Str"("文本.滚动条位置"=w545) -> ()  [unwired: 2 in, 2 out]
        n310 = local read "可乐单价"() -> (w555:dbl)
        n311 = flat-sequence {
          tunnel: [w574] -> w569
          tunnel: w568 -> [w574]
          tunnel: w569 -> [w577]
          frame #0 {
            n312 = Wait (ms)(milliseconds to wait=u32 50) -> ()  [unwired: 1 out]
          }
          frame #1 {
            n313 = property class="Bool (strict)"(reference=w577, "值"=TRUE ("Value")) -> (reference out=w575:refnum<vi>)  [unwired: 1 in, 1 out]
            n314 = Close Reference(reference=w575) -> ()  [unwired: 1 in, 1 out]
          }
        }
        n315 = Add(x=w555, y=w556) -> (x+y=w554:dbl)
        n316 = local write "消费额"(w554) -> ()
        n317 = Get Date/Time String(want seconds? (F)=TRUE) -> (time string=w559:string)  [unwired: 2 in, 1 out]
        n318 = local read "可乐数量"() -> (w566:i32)
        n319 = Concatenate Strings(w559, " " ("string")) -> (w557:string)
        n320 = Get Date/Time String(want seconds? (F)=TRUE) -> (time string=w552:string)  [unwired: 2 in, 1 out]
        n321 = Decrement(x=w566) -> (x-1=w565:i32)
        n322 = Concatenate Strings(w552, " " ("string")) -> (w549:string)
        n323 = local write "可乐数量"(w565) -> ()
        n324 = Concatenate Strings(w563, w557, "可口可乐1罐！" ("出货信息"), "\r") -> (w564:string)
        n325 = Concatenate Strings(w548, w549, "可口可乐1罐！" ("出货信息"), "\r") -> (w546:string)
        n326 = local read "可乐单价"() -> (w567:dbl)
        n327 = Subtract(x=w571, y=w567) -> (x-y=w570:dbl)
      }
      event "王老吉": Value Change {
        n328 = event-data() -> ("CtlRef"=w598:refnum<vi>)  [unwired: 1 in, 5 out]
        n329 = property on="出货信息" class="Str"("文本.滚动条位置"=w578) -> ()  [unwired: 2 in, 2 out]
        n330 = property on="销售记录" class="Str"("文本.滚动条位置"=w578) -> ()  [unwired: 2 in, 2 out]
        n331 = local read "王老吉单价"() -> (w588:dbl)
        n332 = flat-sequence {
          tunnel: [w607] -> w599
          tunnel: w598 -> [w607]
          tunnel: w599 -> [w610]
          frame #0 {
            n333 = Wait (ms)(milliseconds to wait=u32 50) -> ()  [unwired: 1 out]
          }
          frame #1 {
            n334 = property class="Bool (strict)"(reference=w610, "值"=TRUE ("Value")) -> (reference out=w608:refnum<vi>)  [unwired: 1 in, 1 out]
            n335 = Close Reference(reference=w608) -> ()  [unwired: 1 in, 1 out]
          }
        }
        n336 = Add(x=w588, y=w589) -> (x+y=w587:dbl)
        n337 = local write "消费额"(w587) -> ()
        n338 = local read "王老吉数量"() -> (w601:i32)
        n339 = Get Date/Time String(want seconds? (F)=TRUE) -> (time string=w592:string)  [unwired: 2 in, 1 out]
        n340 = Concatenate Strings(w592, " " ("string")) -> (w590:string)
        n341 = Decrement(x=w601) -> (x-1=w600:i32)
        n342 = local write "王老吉数量"(w600) -> ()
        n343 = Get Date/Time String(want seconds? (F)=TRUE) -> (time string=w585:string)  [unwired: 2 in, 1 out]
        n344 = Concatenate Strings(w585, " " ("string")) -> (w582:string)
        n345 = Concatenate Strings(w596, w590, "王老吉1罐！" ("出货信息"), "\r") -> (w597:string)
        n346 = local read "王老吉单价"() -> (w602:dbl)
        n347 = Concatenate Strings(w581, w582, "王老吉1罐！" ("出货信息"), "\r") -> (w580:string)
        n348 = Subtract(x=w604, y=w602) -> (x-y=w603:dbl)
      }
      event "八宝粥": Value Change {
        n349 = event-data() -> ("CtlRef"=w631:refnum<vi>)  [unwired: 1 in, 5 out]
        n350 = property on="出货信息" class="Str"("文本.滚动条位置"=w611) -> ()  [unwired: 2 in, 2 out]
        n351 = property on="销售记录" class="Str"("文本.滚动条位置"=w611) -> ()  [unwired: 2 in, 2 out]
        n352 = flat-sequence {
          tunnel: [w640] -> w632
          tunnel: w631 -> [w640]
          tunnel: w632 -> [w643]
          frame #0 {
            n353 = Wait (ms)(milliseconds to wait=u32 50) -> ()  [unwired: 1 out]
          }
          frame #1 {
            n354 = property class="Bool (strict)"(reference=w643, "值"=TRUE ("Value")) -> (reference out=w641:refnum<vi>)  [unwired: 1 in, 1 out]
            n355 = Close Reference(reference=w641) -> ()  [unwired: 1 in, 1 out]
          }
        }
        n356 = local read "八宝粥单价"() -> (w621:dbl)
        n357 = Add(x=w621, y=w622) -> (x+y=w620:dbl)
        n358 = local write "消费额"(w620) -> ()
        n359 = local read "八宝粥数量"() -> (w634:i32)
        n360 = Get Date/Time String(want seconds? (F)=TRUE) -> (time string=w625:string)  [unwired: 2 in, 1 out]
        n361 = Concatenate Strings(w625, " " ("string")) -> (w623:string)
        n362 = Decrement(x=w634) -> (x-1=w633:i32)
        n363 = local write "八宝粥数量"(w633) -> ()
        n364 = Get Date/Time String(want seconds? (F)=TRUE) -> (time string=w618:string)  [unwired: 2 in, 1 out]
        n365 = Concatenate Strings(w618, " " ("string")) -> (w615:string)
        n366 = Concatenate Strings(w629, w623, "娃哈哈八宝粥1罐！" ("出货信息"), "\r") -> (w630:string)
        n367 = local read "八宝粥单价"() -> (w635:dbl)
        n368 = Concatenate Strings(w614, w615, "娃哈哈八宝粥1罐！" ("出货信息"), "\r") -> (w613:string)
        n369 = Subtract(x=w637, y=w635) -> (x-y=w636:dbl)
      }
      event "红牛": Value Change {
        n370 = event-data() -> ("CtlRef"=w664:refnum<vi>)  [unwired: 1 in, 5 out]
        n371 = property on="出货信息" class="Str"("文本.滚动条位置"=w644) -> ()  [unwired: 2 in, 2 out]
        n372 = property on="销售记录" class="Str"("文本.滚动条位置"=w644) -> ()  [unwired: 2 in, 2 out]
        n373 = flat-sequence {
          tunnel: [w673] -> w665
          tunnel: w664 -> [w673]
          tunnel: w665 -> [w676]
          frame #0 {
            n374 = Wait (ms)(milliseconds to wait=u32 50) -> ()  [unwired: 1 out]
          }
          frame #1 {
            n375 = property class="Bool (strict)"(reference=w676, "值"=TRUE ("Value")) -> (reference out=w674:refnum<vi>)  [unwired: 1 in, 1 out]
            n376 = Close Reference(reference=w674) -> ()  [unwired: 1 in, 1 out]
          }
        }
        n377 = local read "红牛单价"() -> (w654:dbl)
        n378 = Add(x=w654, y=w655) -> (x+y=w653:dbl)
        n379 = local write "消费额"(w653) -> ()
        n380 = local read "红牛数量"() -> (w667:i32)
        n381 = Get Date/Time String(want seconds? (F)=TRUE) -> (time string=w658:string)  [unwired: 2 in, 1 out]
        n382 = Decrement(x=w667) -> (x-1=w666:i32)
        n383 = Concatenate Strings(w658, " " ("string")) -> (w656:string)
        n384 = local write "红牛数量"(w666) -> ()
        n385 = Get Date/Time String(want seconds? (F)=TRUE) -> (time string=w651:string)  [unwired: 2 in, 1 out]
        n386 = Concatenate Strings(w651, " " ("string")) -> (w648:string)
        n387 = Concatenate Strings(w662, w656, "红牛1罐！" ("出货信息"), "\r") -> (w663:string)
        n388 = Concatenate Strings(w647, w648, "红牛1罐！" ("出货信息"), "\r") -> (w646:string)
        n389 = local read "红牛单价"() -> (w668:dbl)
        n390 = Subtract(x=w669, y=w668) -> (x-y=w670:dbl)
      }
      event "雪梨": Value Change {
        n391 = event-data() -> ("CtlRef"=w697:refnum<vi>)  [unwired: 1 in, 5 out]
        n392 = property on="出货信息" class="Str"("文本.滚动条位置"=w677) -> ()  [unwired: 2 in, 2 out]
        n393 = property on="销售记录" class="Str"("文本.滚动条位置"=w677) -> ()  [unwired: 2 in, 2 out]
        n394 = flat-sequence {
          tunnel: [w706] -> w698
          tunnel: w697 -> [w706]
          tunnel: w698 -> [w709]
          frame #0 {
            n395 = Wait (ms)(milliseconds to wait=u32 50) -> ()  [unwired: 1 out]
          }
          frame #1 {
            n396 = property class="Bool (strict)"(reference=w709, "值"=TRUE ("Value")) -> (reference out=w707:refnum<vi>)  [unwired: 1 in, 1 out]
            n397 = Close Reference(reference=w707) -> ()  [unwired: 1 in, 1 out]
          }
        }
        n398 = local read "雪梨单价"() -> (w687:dbl)
        n399 = Add(x=w687, y=w688) -> (x+y=w686:dbl)
        n400 = local read "雪梨数量"() -> (w700:i32)
        n401 = local write "消费额"(w686) -> ()
        n402 = Decrement(x=w700) -> (x-1=w699:i32)
        n403 = Get Date/Time String(want seconds? (F)=TRUE) -> (time string=w691:string)  [unwired: 2 in, 1 out]
        n404 = local write "雪梨数量"(w699) -> ()
        n405 = Concatenate Strings(w691, " " ("string")) -> (w689:string)
        n406 = Get Date/Time String(want seconds? (F)=TRUE) -> (time string=w684:string)  [unwired: 2 in, 1 out]
        n407 = Concatenate Strings(w684, " " ("string")) -> (w681:string)
        n408 = Concatenate Strings(w695, w689, "冰糖雪梨1瓶！" ("出货信息"), "\r") -> (w696:string)
        n409 = local read "雪梨单价"() -> (w701:dbl)
        n410 = Concatenate Strings(w680, w681, "冰糖雪梨1瓶！" ("出货信息"), "\r") -> (w679:string)
        n411 = Subtract(x=w702, y=w701) -> (x-y=w703:dbl)
      }
      event "绿茶": Value Change {
        n412 = event-data() -> ("CtlRef"=w730:refnum<vi>)  [unwired: 1 in, 5 out]
        n413 = property on="出货信息" class="Str"("文本.滚动条位置"=w710) -> ()  [unwired: 2 in, 2 out]
        n414 = property on="销售记录" class="Str"("文本.滚动条位置"=w710) -> ()  [unwired: 2 in, 2 out]
        n415 = flat-sequence {
          tunnel: [w739] -> w731
          tunnel: w730 -> [w739]
          tunnel: w731 -> [w742]
          frame #0 {
            n416 = Wait (ms)(milliseconds to wait=u32 50) -> ()  [unwired: 1 out]
          }
          frame #1 {
            n417 = property class="Bool (strict)"(reference=w742, "值"=TRUE ("Value")) -> (reference out=w740:refnum<vi>)  [unwired: 1 in, 1 out]
            n418 = Close Reference(reference=w740) -> ()  [unwired: 1 in, 1 out]
          }
        }
        n419 = local read "绿茶单价"() -> (w720:dbl)
        n420 = Add(x=w720, y=w721) -> (x+y=w712:dbl)
        n421 = local read "绿茶数量"() -> (w733:i32)
        n422 = local write "消费额"(w712) -> ()
        n423 = Get Date/Time String(want seconds? (F)=TRUE) -> (time string=w724:string)  [unwired: 2 in, 1 out]
        n424 = Decrement(x=w733) -> (x-1=w732:i32)
        n425 = Concatenate Strings(w724, " " ("string")) -> (w722:string)
        n426 = local write "绿茶数量"(w732) -> ()
        n427 = Get Date/Time String(want seconds? (F)=TRUE) -> (time string=w718:string)  [unwired: 2 in, 1 out]
        n428 = Concatenate Strings(w718, " " ("string")) -> (w715:string)
        n429 = Concatenate Strings(w728, w722, "康师傅绿茶1瓶！" ("出货信息"), "\r") -> (w729:string)
        n430 = Concatenate Strings(w714, w715, "康师傅绿茶1瓶！" ("出货信息"), "\r") -> (w713:string)
        n431 = local read "绿茶单价"() -> (w734:dbl)
        n432 = Subtract(x=w735, y=w734) -> (x-y=w737:dbl)
      }
      event "花生奶": Value Change {
        n433 = event-data() -> ("CtlRef"=w763:refnum<vi>)  [unwired: 1 in, 5 out]
        n434 = property on="出货信息" class="Str"("文本.滚动条位置"=w743) -> ()  [unwired: 2 in, 2 out]
        n435 = property on="销售记录" class="Str"("文本.滚动条位置"=w743) -> ()  [unwired: 2 in, 2 out]
        n436 = flat-sequence {
          tunnel: [w772] -> w764
          tunnel: w763 -> [w772]
          tunnel: w764 -> [w775]
          frame #0 {
            n437 = Wait (ms)(milliseconds to wait=u32 50) -> ()  [unwired: 1 out]
          }
          frame #1 {
            n438 = property class="Bool (strict)"(reference=w775, "值"=TRUE ("Value")) -> (reference out=w773:refnum<vi>)  [unwired: 1 in, 1 out]
            n439 = Close Reference(reference=w773) -> ()  [unwired: 1 in, 1 out]
          }
        }
        n440 = local read "花生奶单价"() -> (w753:dbl)
        n441 = Add(x=w753, y=w754) -> (x+y=w752:dbl)
        n442 = local read "花生奶数量"() -> (w766:i32)
        n443 = Get Date/Time String(want seconds? (F)=TRUE) -> (time string=w757:string)  [unwired: 2 in, 1 out]
        n444 = local write "消费额"(w752) -> ()
        n445 = Concatenate Strings(w757, " " ("string")) -> (w755:string)
        n446 = Decrement(x=w766) -> (x-1=w765:i32)
        n447 = local write "花生奶数量"(w765) -> ()
        n448 = Get Date/Time String(want seconds? (F)=TRUE) -> (time string=w750:string)  [unwired: 2 in, 1 out]
        n449 = Concatenate Strings(w761, w755, "银鹭花生奶1瓶！" ("出货信息"), "\r") -> (w762:string)
        n450 = Concatenate Strings(w750, " " ("string")) -> (w747:string)
        n451 = local read "花生奶单价"() -> (w767:dbl)
        n452 = Concatenate Strings(w746, w747, "银鹭花生奶1瓶！" ("出货信息"), "\r") -> (w745:string)
        n453 = Subtract(x=w768, y=w767) -> (x-y=w769:dbl)
      }
      event "矿泉水": Value Change {
        n454 = event-data() -> ("CtlRef"=w796:refnum<vi>)  [unwired: 1 in, 5 out]
        n455 = property on="出货信息" class="Str"("文本.滚动条位置"=w776) -> ()  [unwired: 2 in, 2 out]
        n456 = property on="销售记录" class="Str"("文本.滚动条位置"=w776) -> ()  [unwired: 2 in, 2 out]
        n457 = flat-sequence {
          tunnel: [w805] -> w797
          tunnel: w796 -> [w805]
          tunnel: w797 -> [w808]
          frame #0 {
            n458 = Wait (ms)(milliseconds to wait=u32 50) -> ()  [unwired: 1 out]
          }
          frame #1 {
            n459 = property class="Bool (strict)"(reference=w808, "值"=TRUE ("Value")) -> (reference out=w806:refnum<vi>)  [unwired: 1 in, 1 out]
            n460 = Close Reference(reference=w806) -> ()  [unwired: 1 in, 1 out]
          }
        }
        n461 = local read "矿泉水单价"() -> (w786:dbl)
        n462 = Add(x=w786, y=w787) -> (x+y=w785:dbl)
        n463 = local write "消费额"(w785) -> ()
        n464 = local read "矿泉水数量"() -> (w799:i32)
        n465 = Get Date/Time String(want seconds? (F)=TRUE) -> (time string=w790:string)  [unwired: 2 in, 1 out]
        n466 = Concatenate Strings(w790, " " ("string")) -> (w788:string)
        n467 = Decrement(x=w799) -> (x-1=w798:i32)
        n468 = local write "矿泉水数量"(w798) -> ()
        n469 = Get Date/Time String(want seconds? (F)=TRUE) -> (time string=w783:string)  [unwired: 2 in, 1 out]
        n470 = Concatenate Strings(w783, " " ("string")) -> (w780:string)
        n471 = Concatenate Strings(w794, w788, "怡宝矿泉水1瓶！" ("出货信息"), "\r") -> (w795:string)
        n472 = local read "矿泉水单价"() -> (w801:dbl)
        n473 = Concatenate Strings(w779, w780, "怡宝矿泉水1瓶！" ("出货信息"), "\r") -> (w778:string)
        n474 = Subtract(x=w802, y=w801) -> (x-y=w803:dbl)
      }
      event "营养快线": Value Change {
        n475 = event-data() -> ("CtlRef"=w829:refnum<vi>)  [unwired: 1 in, 5 out]
        n476 = property on="出货信息" class="Str"("文本.滚动条位置"=w809) -> ()  [unwired: 2 in, 2 out]
        n477 = property on="销售记录" class="Str"("文本.滚动条位置"=w809) -> ()  [unwired: 2 in, 2 out]
        n478 = flat-sequence {
          tunnel: [w838] -> w830
          tunnel: w829 -> [w838]
          tunnel: w830 -> [w841]
          frame #0 {
            n479 = Wait (ms)(milliseconds to wait=u32 50) -> ()  [unwired: 1 out]
          }
          frame #1 {
            n480 = property class="Bool (strict)"(reference=w841, "值"=TRUE ("Value")) -> (reference out=w839:refnum<vi>)  [unwired: 1 in, 1 out]
            n481 = Close Reference(reference=w839) -> ()  [unwired: 1 in, 1 out]
          }
        }
        n482 = local read "营养快线单价"() -> (w819:dbl)
        n483 = Add(x=w819, y=w820) -> (x+y=w818:dbl)
        n484 = local read "营养快线数量"() -> (w832:i32)
        n485 = Get Date/Time String(want seconds? (F)=TRUE) -> (time string=w823:string)  [unwired: 2 in, 1 out]
        n486 = local write "消费额"(w818) -> ()
        n487 = Concatenate Strings(w823, " " ("string")) -> (w821:string)
        n488 = Decrement(x=w832) -> (x-1=w831:i32)
        n489 = Get Date/Time String(want seconds? (F)=TRUE) -> (time string=w816:string)  [unwired: 2 in, 1 out]
        n490 = local write "营养快线数量"(w831) -> ()
        n491 = Concatenate Strings(w816, " " ("string")) -> (w813:string)
        n492 = Concatenate Strings(w827, w821, "娃哈哈营养快线1瓶！" ("出货信息"), "\r") -> (w828:string)
        n493 = Concatenate Strings(w812, w813, "娃哈哈营养快线1瓶！" ("出货信息"), "\r") -> (w811:string)
        n494 = local read "营养快线单价"() -> (w833:dbl)
        n495 = Subtract(x=w834, y=w833) -> (x-y=w835:dbl)
      }
      event "果粒橙": Value Change {
        n496 = event-data() -> ("CtlRef"=w862:refnum<vi>)  [unwired: 1 in, 5 out]
        n497 = property on="出货信息" class="Str"("文本.滚动条位置"=w842) -> ()  [unwired: 2 in, 2 out]
        n498 = property on="销售记录" class="Str"("文本.滚动条位置"=w842) -> ()  [unwired: 2 in, 2 out]
        n499 = flat-sequence {
          tunnel: [w871] -> w863
          tunnel: w862 -> [w871]
          tunnel: w863 -> [w874]
          frame #0 {
            n500 = Wait (ms)(milliseconds to wait=u32 50) -> ()  [unwired: 1 out]
          }
          frame #1 {
            n501 = property class="Bool (strict)"(reference=w874, "值"=TRUE ("Value")) -> (reference out=w872:refnum<vi>)  [unwired: 1 in, 1 out]
            n502 = Close Reference(reference=w872) -> ()  [unwired: 1 in, 1 out]
          }
        }
        n503 = local read "果粒橙单价"() -> (w852:dbl)
        n504 = Add(x=w852, y=w853) -> (x+y=w851:dbl)
        n505 = local write "消费额"(w851) -> ()
        n506 = local read "果粒橙数量"() -> (w865:i32)
        n507 = Get Date/Time String(want seconds? (F)=TRUE) -> (time string=w856:string)  [unwired: 2 in, 1 out]
        n508 = Concatenate Strings(w856, " " ("string")) -> (w854:string)
        n509 = Decrement(x=w865) -> (x-1=w864:i32)
        n510 = Get Date/Time String(want seconds? (F)=TRUE) -> (time string=w849:string)  [unwired: 2 in, 1 out]
        n511 = local write "果粒橙数量"(w864) -> ()
        n512 = Concatenate Strings(w849, " " ("string")) -> (w846:string)
        n513 = Concatenate Strings(w860, w854, "美之源果粒橙1瓶！" ("出货信息"), "\r") -> (w861:string)
        n514 = Concatenate Strings(w845, w846, "美之源果粒橙1瓶！" ("出货信息"), "\r") -> (w844:string)
        n515 = local read "果粒橙单价"() -> (w866:dbl)
        n516 = Subtract(x=w868, y=w866) -> (x-y=w867:dbl)
      }
      event "上货": Value Change {
        n517 = event-data() -> ("CtlRef"=w878:refnum<vi>)  [unwired: 1 in, 5 out]
        n518 = flat-sequence {
          tunnel: [w889] -> w877
          tunnel: w875 -> [w888]
          frame #0 {
            w892 = "  ;  " ("string")
            w941 = 20 ("百事数量")
            n519 = local read "百事数量"() -> (w953:i32)
            n520 = local read "可乐数量"() -> (w952:i32)
            n521 = local read "花生奶数量"() -> (w951:i32)
            n522 = local read "王老吉数量"() -> (w950:i32)
            n523 = local read "八宝粥数量"() -> (w949:i32)
            n524 = local read "红牛数量"() -> (w948:i32)
            n525 = local read "雪梨数量"() -> (w947:i32)
            n526 = local read "果粒橙数量"() -> (w946:i32)
            n527 = local read "矿泉水数量"() -> (w945:i32)
            n528 = local read "绿茶数量"() -> (w944:i32)
            n529 = local read "营养快线数量"() -> (w943:i32)
            n530 = local read "雪碧数量"() -> (w942:i32)
            n531 = Subtract(x=w941, y=w953) -> (x-y=w940:i32)
            n532 = Subtract(x=w941, y=w952) -> (x-y=w939:i32)
            n533 = Subtract(x=w941, y=w951) -> (x-y=w938:i32)
            n534 = Subtract(x=w941, y=w950) -> (x-y=w937:i32)
            n535 = Subtract(x=w941, y=w949) -> (x-y=w936:i32)
            n536 = Subtract(x=w941, y=w948) -> (x-y=w935:i32)
            n537 = Subtract(x=w941, y=w947) -> (x-y=w934:i32)
            n538 = Subtract(x=w941, y=w946) -> (x-y=w933:i32)
            n539 = Subtract(x=w941, y=w945) -> (x-y=w932:i32)
            n540 = Subtract(x=w941, y=w944) -> (x-y=w931:i32)
            n541 = Subtract(x=w941, y=w943) -> (x-y=w930:i32)
            n542 = Subtract(x=w941, y=w942) -> (x-y=w929:i32)
            n543 = Number To Decimal String(number=w940) -> (decimal integer string=w927:string)  [unwired: 1 in]
            n544 = Number To Decimal String(number=w939) -> (decimal integer string=w915:string)  [unwired: 1 in]
            n545 = Number To Decimal String(number=w938) -> (decimal integer string=w914:string)  [unwired: 1 in]
            n546 = Number To Decimal String(number=w937) -> (decimal integer string=w913:string)  [unwired: 1 in]
            n547 = Number To Decimal String(number=w936) -> (decimal integer string=w912:string)  [unwired: 1 in]
            n548 = Number To Decimal String(number=w935) -> (decimal integer string=w911:string)  [unwired: 1 in]
            n549 = Number To Decimal String(number=w934) -> (decimal integer string=w910:string)  [unwired: 1 in]
            n550 = Number To Decimal String(number=w933) -> (decimal integer string=w909:string)  [unwired: 1 in]
            n551 = Number To Decimal String(number=w932) -> (decimal integer string=w908:string)  [unwired: 1 in]
            n552 = Number To Decimal String(number=w931) -> (decimal integer string=w907:string)  [unwired: 1 in]
            n553 = Number To Decimal String(number=w930) -> (decimal integer string=w906:string)  [unwired: 1 in]
            n554 = Number To Decimal String(number=w929) -> (decimal integer string=w905:string)  [unwired: 1 in]
            n555 = Get Date/Time String(want seconds? (F)=TRUE) -> (time string=w886:string)  [unwired: 2 in, 1 out]
            n556 = Concatenate Strings(w886, " " ("string")) -> (w884:string)
            n557 = Concatenate Strings("百事+" ("string"), w927) -> (w903:string)
            n558 = Concatenate Strings("可乐+" ("string"), w915) -> (w902:string)
            n559 = Concatenate Strings("花生奶+" ("string"), w914) -> (w901:string)
            n560 = Concatenate Strings("王老吉+" ("string"), w913) -> (w900:string)
            n561 = Concatenate Strings("八宝粥+" ("string"), w912) -> (w899:string)
            n562 = Concatenate Strings("红牛+" ("string"), w911) -> (w898:string)
            n563 = Concatenate Strings("雪梨+" ("string"), w910) -> (w897:string)
            n564 = Concatenate Strings("果粒橙+" ("string"), w909) -> (w896:string)
            n565 = Concatenate Strings("矿泉水+" ("string"), w908) -> (w895:string)
            n566 = Concatenate Strings("绿茶+" ("string"), w907) -> (w894:string)
            n567 = Concatenate Strings("营养快线+" ("string"), w906) -> (w893:string)
            n568 = Concatenate Strings("雪碧+" ("string"), w905) -> (w891:string)
            n569 = Concatenate Strings(w888, w884, "上货信息:" ("string"), w903, w892, w902, w892, w901, w892, w900, w892, w899, w892, w898, w892, w897, w892, w896, w892, w895, w892, w894, w892, w893, w892, w891, "\r") -> (w889:string)
          }
          frame #1 {
            w954 = 20 ("百事数量")
            n570 = local write "百事数量"(w954) -> ()
            n571 = local write "可乐数量"(w954) -> ()
            n572 = local write "花生奶数量"(w954) -> ()
            n573 = local write "王老吉数量"(w954) -> ()
            n574 = local write "八宝粥数量"(w954) -> ()
            n575 = local write "红牛数量"(w954) -> ()
            n576 = local write "雪梨数量"(w954) -> ()
            n577 = local write "果粒橙数量"(w954) -> ()
            n578 = local write "矿泉水数量"(w954) -> ()
            n579 = local write "绿茶数量"(w954) -> ()
            n580 = local write "营养快线数量"(w954) -> ()
            n581 = local write "雪碧数量"(w954) -> ()
          }
        }
        n582 = property on="销售记录" class="Str"("文本.滚动条位置"=w876) -> ()  [unwired: 2 in, 2 out]
        n583 = flat-sequence {
          tunnel: [w956] -> w879
          tunnel: w878 -> [w956]
          tunnel: w879 -> [w959]
          frame #0 {
            n584 = Wait (ms)(milliseconds to wait=u32 50) -> ()  [unwired: 1 out]
          }
          frame #1 {
            n585 = property class="Bool (strict)"(reference=w959, "值"=FALSE ("Value")) -> (reference out=w957:refnum<vi>)  [unwired: 1 in, 1 out]
            n586 = Close Reference(reference=w957) -> ()  [unwired: 1 in, 1 out]
          }
        }
      }
    }
    n587 = local read "营养快线单价"() -> (w34:dbl)
    n588 = local read "矿泉水单价"() -> (w25:dbl)
    n589 = local read "花生奶单价"() -> (w22:dbl)
    n590 = local read "果粒橙单价"() -> (w37:dbl)
    n591 = local write "投币金额"(w92) -> ()
    n592 = Round Toward -Infinity(1:w92) -> (0:w90:dbl)
    n593 = Round Toward -Infinity(1:w10) -> (0:w14:dbl)
    n594 = Subtract(x=w92, y=w90) -> (x-y=w94:dbl)
    n595 = Subtract(x=w10, y=w14) -> (x-y=w12:dbl)
    n596 = Equal?(x=w94, y=0.5) -> (x = y?=w93:bool)
    n597 = Round Toward -Infinity(1:w25) -> (0:w29:dbl)
    n598 = Round Toward -Infinity(1:w22) -> (0:w18:dbl)
    n599 = Round Toward -Infinity(1:w34) -> (0:w30:dbl)
    n600 = Round Toward -Infinity(1:w37) -> (0:w41:dbl)
    n601 = Equal?(x=w12, y=0.5) -> (x = y?=w13:bool)
    n602 = Subtract(x=w25, y=w29) -> (x-y=w27:dbl)
    n603 = Subtract(x=w22, y=w18) -> (x-y=w20:dbl)
    n604 = Subtract(x=w34, y=w30) -> (x-y=w32:dbl)
    n605 = Subtract(x=w37, y=w41) -> (x-y=w39:dbl)
    n606 = case shown="真" w93 {
      tunnel: w90 -> [w204 w209]
      tunnel: [w203 w207] -> w91
      frame False {
        n607 = Number To Decimal String(number=w204) -> (decimal integer string=w205:string)  [unwired: 1 in]
        n608 = Concatenate Strings(w205, "元" ("string")) -> (w203:string)
      }
      frame True {
        n609 = Number To Decimal String(number=w209) -> (decimal integer string=w210:string)  [unwired: 1 in]
        n610 = Concatenate Strings(w210, ".5元" ("string")) -> (w207:string)
      }
    }
    n611 = Equal?(x=w27, y=0.5) -> (x = y?=w28:bool)
    n612 = Equal?(x=w20, y=0.5) -> (x = y?=w19:bool)
    n613 = Equal?(x=w32, y=0.5) -> (x = y?=w31:bool)
    n614 = Equal?(x=w39, y=0.5) -> (x = y?=w40:bool)
    n615 = case shown="假" w13 {
      tunnel: w14 -> [w100 w105]
      tunnel: [w99 w103] -> w9
      frame False {
        n616 = Number To Decimal String(number=w100) -> (decimal integer string=w101:string)  [unwired: 1 in]
        n617 = Concatenate Strings(w101, "元" ("string")) -> (w99:string)
      }
      frame True {
        n618 = Number To Decimal String(number=w105) -> (decimal integer string=w106:string)  [unwired: 1 in]
        n619 = Concatenate Strings(w106, ".5元" ("string")) -> (w103:string)
      }
    }
    n620 = case shown="真" w28 {
      tunnel: w29 -> [w124 w129]
      tunnel: [w123 w127] -> w24
      frame False {
        n621 = Number To Decimal String(number=w124) -> (decimal integer string=w125:string)  [unwired: 1 in]
        n622 = Concatenate Strings(w125, "元" ("string")) -> (w123:string)
      }
      frame True {
        n623 = Number To Decimal String(number=w129) -> (decimal integer string=w130:string)  [unwired: 1 in]
        n624 = Concatenate Strings(w130, ".5元" ("string")) -> (w127:string)
      }
    }
    n625 = case shown="真" w19 {
      tunnel: w18 -> [w132 w137]
      tunnel: [w131 w135] -> w23
      frame False {
        n626 = Number To Decimal String(number=w132) -> (decimal integer string=w133:string)  [unwired: 1 in]
        n627 = Concatenate Strings(w133, "元" ("string")) -> (w131:string)
      }
      frame True {
        n628 = Number To Decimal String(number=w137) -> (decimal integer string=w138:string)  [unwired: 1 in]
        n629 = Concatenate Strings(w138, ".5元" ("string")) -> (w135:string)
      }
    }
    n630 = case shown="真" w31 {
      tunnel: w30 -> [w116 w121]
      tunnel: [w115 w119] -> w35
      frame False {
        n631 = Number To Decimal String(number=w116) -> (decimal integer string=w117:string)  [unwired: 1 in]
        n632 = Concatenate Strings(w117, "元" ("string")) -> (w115:string)
      }
      frame True {
        n633 = Number To Decimal String(number=w121) -> (decimal integer string=w122:string)  [unwired: 1 in]
        n634 = Concatenate Strings(w122, ".5元" ("string")) -> (w119:string)
      }
    }
    n635 = local write "出货信息"(w17) -> ()
    n636 = local write "销售记录"(w7) -> ()
    n637 = case shown="真" w40 {
      tunnel: w41 -> [w108 w113]
      tunnel: [w107 w111] -> w36
      frame False {
        n638 = Number To Decimal String(number=w108) -> (decimal integer string=w109:string)  [unwired: 1 in]
        n639 = Concatenate Strings(w109, "元" ("string")) -> (w107:string)
      }
      frame True {
        n640 = Number To Decimal String(number=w113) -> (decimal integer string=w114:string)  [unwired: 1 in]
        n641 = Concatenate Strings(w114, ".5元" ("string")) -> (w111:string)
      }
    }
    n642 = local write "显示金额"(w91) -> ()
    n643 = local write "销售金额"(w9) -> ()
    n644 = local write "营养快线P"(w35) -> ()
    n645 = local write "矿泉水P"(w24) -> ()
    n646 = local write "花生奶P"(w23) -> ()
    n647 = local write "果粒橙P"(w36) -> ()
  }
